vi "Load Hot Pixel Map.vi"(8 "Error In":errorcluster, 9 "Verbose (F)":bool, 11 "Hot Pixel Mask Image Path":path) -> (0 "Error Out":errorcluster, 3 "Mask Image Dimensions":i32[](array[numeric]))   [LabVIEW 2021]
uses:
  <vilib>/Utility/error.llb/DialogType.ctl
  SwissSPAD/SwissSPAD Live_Image Display Options.ctl
  SwissSPAD/SwissSPAD Live_Settings List.ctl
  Notebook/Notebook.lvlib
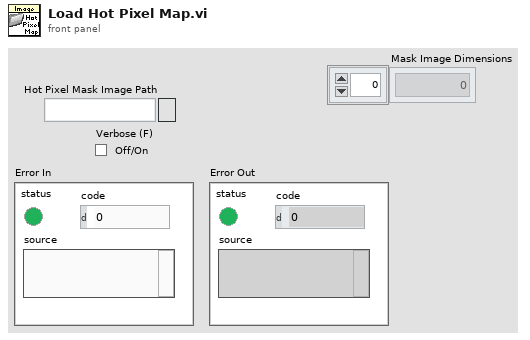
[diagram p1: front panel]
types:
  T1 = typedef "SwissSPAD Live_Settings List.ctl" = enum16{"FPGA:Bottom Half", "FPGA:Top Half", "FPGA:Bottom Bitfile Path", "FPGA:Top Bitfile Path", "FPGA:Bottom Bitstream Version", "FPGA:Top Bitstream Version", "FPGA:Auto Reset FPGA", "FPGA:Bottom FPGA Serial Number", "FPGA:Top FPGA Serial Number", "FPGA:Detector PCB Version", "Acquisition Parameters:Microlens", "Acquisition Parameters:SS2 DAQ Parameters", "Acquisition Parameters:Gate Configuration Array", "Acquisition Parameters:SS3 DAQ Parameters", "Acquisition Parameters:Buffer Size (# 8-bit Gates)", "File Information:File Information", "File Information:# Datasets in Series", "File Information:Scrambled File Flag", "File Information:SS3 Gate Slip Correction", "File Information:SS3 Hot Pixel Mismatch Detection", "File Information:Delay between Datasets", "File Information:Save Sum of All Gates Preview", "Image Parameters:Image ROI Information", "Image Parameters:Image Binning Options", "Image Parameters:SS3 Displayed Image", "Image Parameters:Image Display Options", "Image Parameters:Use Histogram Cursors", "Image Parameter:FPGA Data to Display", "UI Settings:Histogram Bins Number", "UI Settings:Histogram Bin Size", "UI Settings:Use Image Display Options", "UI Settings:Verbose Settings", "UI Settings:Verbose Saving"}
  T2 = typedef "SwissSPAD Live_Image Display Options.ctl" = cluster{"Remove Screamers":bool, "Delta":sgl, "Equalize Histogram":bool, "Percentile":sgl, "Hot Pixel Mask Image":path, "Use Hot Pixel Mask":bool}
  T3 = typedef "Image Type" = u32
  T4 = typedef "IMAQ Image.ctl" = refnum<image>
  T5 = typedef "DialogType.ctl" = u16
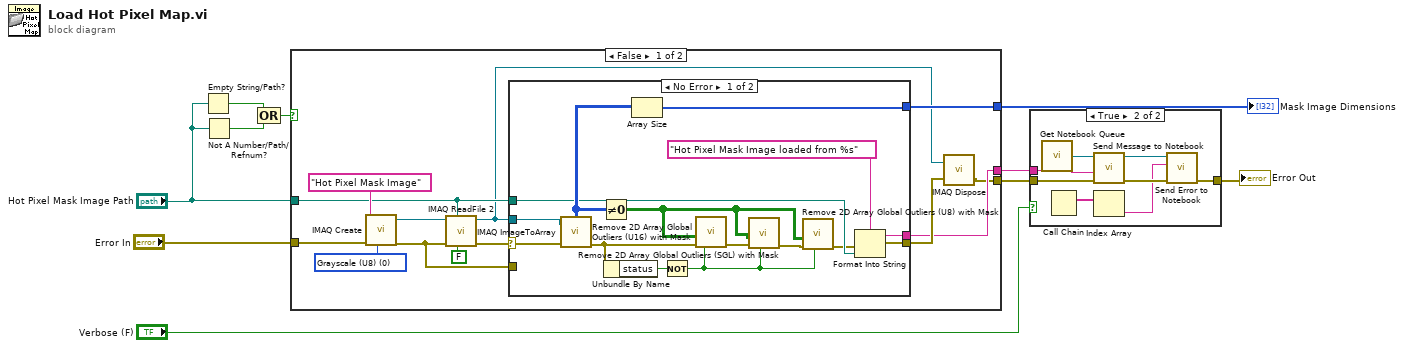
[diagram p0: block diagram]
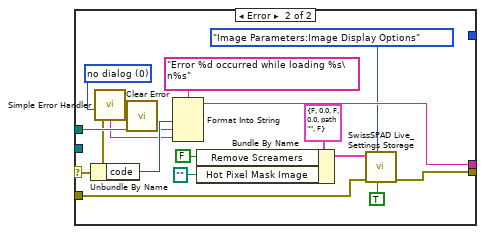
[diagram p3: hidden frame]
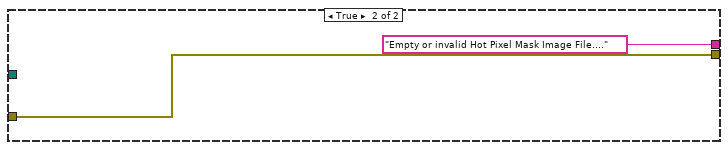
[diagram p4: hidden frame]
diagram:
  n1 = Empty String/Path?(string/path="Hot Pixel Mask Image Path") -> (empty?=w5:bool)
  n2 = Not A Number/Path/Refnum?(number/path/refnum="Hot Pixel Mask Image Path") -> (NaN/Path/Refnum?=w4:bool)
  n3 = Compound Arithmetic op=OR(w5, w4) -> (w3:bool)
  n4 = case shown="False" w3 {
    tunnel: "Error In" -> [w21 w56]
    tunnel: [w13 w56] -> w9
    tunnel: [w14 "Empty or invalid Hot Pixel Mask Image File...."] -> w8
    tunnel: "Hot Pixel Mask Image Path" -> [w15 _]
    tunnel: [w17 _] -> w2
    frame False {
      w22 = T3 0 items=["Grayscale (U8)", "Grayscale (I16)", "Grayscale (SGL)", "Complex (CSG)", "RGB (U32)", "HSL (U32)", "RGB (U64)", "Grayscale (U16)"] ("Image Type")
      n5 = call "IMAQ Create"("Image Name"="Hot Pixel Mask Image", "Image Type"=w22, "error in (no error)"=w21) -> ("New Image"=w20:T4, "error out"=w11:errorcluster)  [unwired: 2 in]
      n6 = call "IMAQ ReadFile 2"("Use File Path Image Type"=FALSE, "File Path"=w15, "error in (no error)"=w11, "Image"=w20) -> ("error out"=w18:errorcluster, "Image Out"=w12:T4)  [unwired: 3 in, 3 out]
      n7 = case shown="No Error" w18 {
        selector: w18 -> [w38 w50]
        tunnel: w12 -> [w35 _]
        tunnel: [w32 _] -> w17
        tunnel: [w24 w41] -> w16
        tunnel: w15 -> [w28 w53]
        tunnel: [w27 w52] -> w14
        tunnel: w11 -> [_ w42]
        frame No Error {
          n8 = call "IMAQ ImageToArray"("error in (no error)"=w38, "Image"=w35) -> ("error out"=w37:errorcluster, "Image Pixels (U8)"=w33:u8[][])  [unwired: 2 in, 3 out]
          n9 = Not Equal To 0?(x=w33) -> (x != 0?=w30:bool[][])
          n10 = Unbundle By Name(w37) -> ("status"=w36:bool)
          n11 = Array Size(array=w33) -> (size(s)=w32:i32[])
          n12 = Not(x=w36) -> (.not. x?=w29:bool)
          n13 = call "Remove 2D Array Global Outliers (U16) with Mask.vi"("Init?"=w29, "Error In"=w37, "2D Mask in"=w30) -> ("Error Out"=w34:errorcluster)  [unwired: 5 in, 3 out]
          n14 = call "Remove 2D Array Global Outliers (SGL) with Mask.vi"("Init?"=w29, "Error In"=w34, "2D Mask in"=w30) -> ("Error Out"=w31:errorcluster)  [unwired: 6 in, 2 out]
          n15 = call "Remove 2D Array Global Outliers (U8) with Mask.vi"("Init?"=w29, "Error In"=w31, "2D Mask in"=w30) -> ("Error Out"=w26:errorcluster)  [unwired: 5 in, 3 out]
          n16 = Format Into String(format string="Hot Pixel Mask Image loaded from %s", error in=w26, w28) -> (resulting string=w27:string, error out=w24:errorcluster)  [unwired: 1 in]
        }
        frame Error {
          w47 = T5 0 items=["no dialog", "OK message", "continue or stop message", "OK message + warnings", "continue/stop + warnings"] ("type of dialog (OK msg:1)")
          n17 = Unbundle By Name(w50) -> ("code"=w54:i32)
          n18 = call <vilib>:"Simple Error Handler.vi"("type of dialog (OK msg:1)"=w47, "error in (no error)"=w50) -> ("error out"=w48:errorcluster, "message"=w49:string)  [unwired: 3 in, 3 out]
          n19 = call "Clear Error.vi"("Error In"=w48) -> ()  [unwired: 8 in, 1 out]
          n20 = Format Into String(format string="Error %d occurred while loading %s\n%s", w54, w53, w49) -> (resulting string=w52:string)  [unwired: 2 in, 1 out]
          n21 = Bundle By Name(cluster=T2 {"Remove Screamers"=FALSE, "Delta"=0.0, "Equalize Histogram"=FALSE, "Percentile"=0.0, "Hot Pixel Mask Image"=path "", "Use Hot Pixel Mask"=FALSE} ("Image Display Options"), "Remove Screamers"=FALSE, "Hot Pixel Mask Image"=path "") -> (w46:T2)
          n22 = call "SwissSPAD Live_Settings Storage.vi"("Set/Get(F)"=TRUE, "Settings List"=SwissSPAD_Live_Settings_List."Image Parameters:Image Display Options", "Error In"=w42, "Variant Data in"=w46) -> ("Error Out"=w41:errorcluster)  [unwired: 6 in, 1 out]
        }
      }
      n23 = call "IMAQ Dispose"("Image"=w12, "error in (no error)"=w16) -> ("error out"=w13:errorcluster)  [unwired: 4 in]
    }
    frame True {
    }
  }
  "Mask Image Dimensions" <- w2
  n24 = case shown="True" "Verbose (F)" {
    tunnel: w9 -> [w57 w65]
    tunnel: w8 -> [_ w64]
    tunnel: [w57 w61] -> w7
    frame False {
    }
    frame True {
      n25 = call "Get Notebook Queue.vi"() -> ("Notebook Queue"=w63:refnum<queue>)  [unwired: 9 in]
      n26 = Call Chain() -> (call chain=w59:string[])
      n27 = call "Send Message to Notebook.vi"("Error In"=w65, "Message"=w64, "Notebook Queue"=w63) -> ("Error Out"=w62:errorcluster, "Notebook Queue"=w60:refnum<queue>)  [unwired: 5 in]
      n28 = Index Array(array=w59) -> (element=w58:string)  [unwired: 1 in]
      n29 = call "Send Error to Notebook.vi"("error in (no error)"=w62, "State Machine Case Error Source"=w58, "Notebook Q"=w60) -> ("Error Out"=w61:errorcluster)  [unwired: 8 in]
    }
  }
  "Error Out" <- w7
